vi "Save Snap.vi"() -> (3 "Image Out":T1(plugin-control))   [LabVIEW 2013]
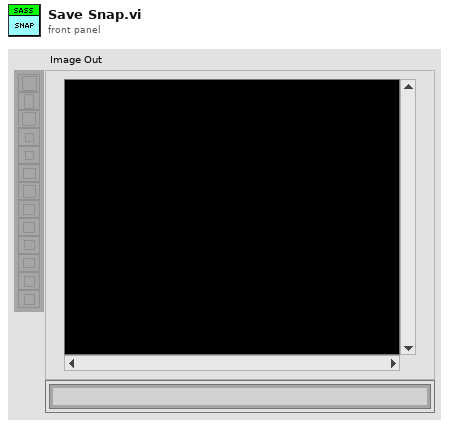
[diagram p1: front panel]
types:
  T1 = typedef "IMAQ Image.ctl" = refnum<image>
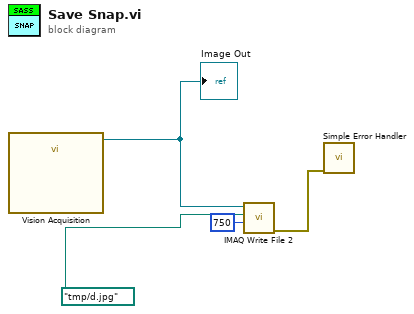
[diagram p0: block diagram]
diagram:
  n1 = call "Vision Acquisition"() -> ("Image Out"=w1:T1)  [unwired: 26 in, 1 out]
  "Image Out" <- w1
  n2 = call-poly "IMAQ Write File 2"("Image Quality"=u32 750, "File Path"=path "/tmp/d.jpg", "Image"=w1) -> ("error out"=w2:errorcluster)  [unwired: 7 in, 1 out]
  n3 = call <vilib>:"Simple Error Handler.vi"("error in (no error)"=w2) -> ()  [unwired: 4 in, 5 out]
